vi "ReceiveCallbackVI.vi"(4 "queue out":refnum<queue>, 5 "Event Data":cluster{"sender":refnum<k24>, "e":refnum<k24>}, 6 "Control Ref":refnum<k24>, 7 "Event Common Data":T1) -> ()   [LabVIEW 2018]
uses:
  C:/Users/chrismadlax/Desktop/LVSampleCode/dotNETCallback/netstandard2.0/myClass2.dll
  netstandard2.0/myClass2.dll
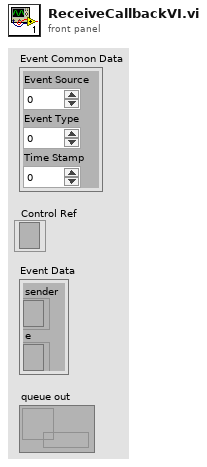
[diagram p1: front panel]
types:
  T1 = cluster{"Event Source":i32, "Event Type":u32, "Time Stamp":u32}
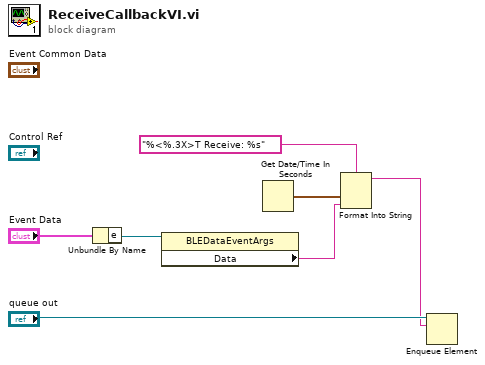
[diagram p0: block diagram]
diagram:
  n1 = Unbundle By Name("Event Data") -> ("e"=w5:refnum<k24>)
  n2 = property class="BLEDataEventArgs"(reference=w5) -> ("Data"=w2:string)  [unwired: 1 in, 2 out]
  n3 = Get Date/Time In Seconds() -> (seconds since 1Jan1904=w3:timestamp)
  n4 = Format Into String(format string="%<%.3X>T Receive: %s", w3, w2) -> (resulting string=w1:string)  [unwired: 2 in, 1 out]
  n5 = Enqueue Element(queue="queue out", element=w1) -> ()  [unwired: 2 in, 3 out]
